vi "Gather Samples.vi"(8 "error in (no error)":errorcluster, 11 "Transfer Line in":refnum<class "Transfer Line.lvclass">) -> (0 "error out":errorcluster, 2 "Samples":refnum<class "Sample.lvclass">[](array[class]), 3 "Transfer Line out":refnum<class "Transfer Line.lvclass">)   [LabVIEW 2015, in "cRIO-Carbondioxide.lvlib" / "CO2-Actor.lvlib" / "Transfer Line.lvclass"]
uses:
  Transfer Line.lvclass
  subs/Sample/Sample.lvclass
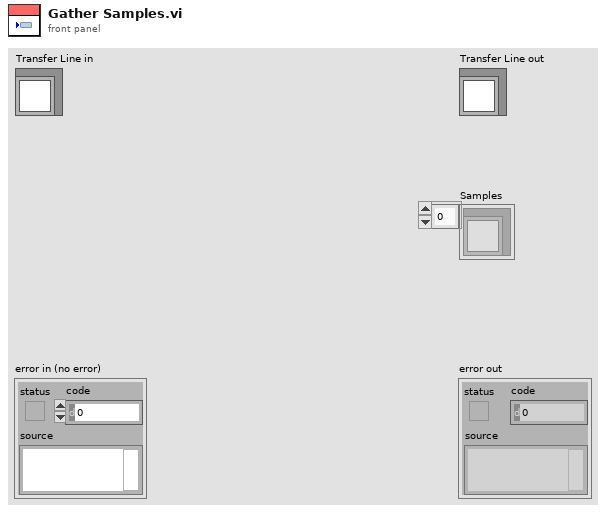
[diagram p1: front panel]
types:
  T1 = enum16{"None", "Sample Line", "Storage Line", "Syringe", "Preparation Line", "Transfer Line", "He Line"}[]
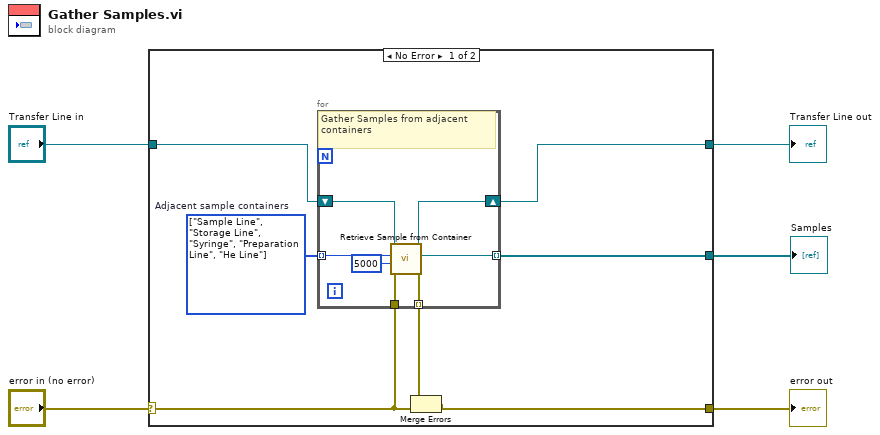
[diagram p0: block diagram]
diagram:
  n1 = case shown="No Error" "error in (no error)" {
    selector: "error in (no error)" -> [w7 w21]
    tunnel: [w6 w21] -> w3
    tunnel: [w8 w20] -> w4
    tunnel: "Transfer Line in" -> [w10 w20]
    tunnel: [w9 _] -> w1
    frame No Error {
      w12 = T1 [enum."Sample Line", enum."Storage Line", enum."Syringe", enum."Preparation Line", enum."He Line"] items=["None", "Sample Line", "Storage Line", "Syringe", "Preparation Line", "Transfer Line", "He Line"]  # Adjacent sample containers
      n2 = for {
        tunnel: w7 -> [w19]
        tunnel: [w18] -> w11 mode=indexing
        tunnel: w12 -> [w17] mode=indexing
        tunnel: [w16] -> w9 mode=indexing
        shift-right: [w15] -> w8
        shift-left: w10 -> [w14]
        # "Gather Samples from adjacent containers"
        n3 = call "Retrieve Sample from Container.vi"("error in (no error)"=w19, "timeout in ms (1000)"=5000, "Container"=w17, "Transfer Line in"=w14) -> ("error out"=w18:errorcluster, "Sample out"=w16:refnum<class "Sample.lvclass">, "Transfer Line out"=w15:refnum<class "Transfer Line.lvclass">)  [unwired: 5 in]
      }
      n4 = Merge Errors(w11, w7) -> (w6:errorcluster)
    }
    frame Error {
    }
  }
  "error out" <- w3
  "Transfer Line out" <- w4
  "Samples" <- w1
